vi "PH_Timing.Update GUI.vi"(0 "i ref in":refnum<vi>, 5 "error in (no error)":errorcluster) -> (14 "i ref out":refnum<vi>, 19 "error out":errorcluster)   [LabVIEW 2014, in "PH_Timing.lvlib"]
doc: "By this VI several the blinking of several GUI elements is set which is depending on some information."
uses:
  PH_Timing.lvlib
  PH_Common/PH_Common.lvlib
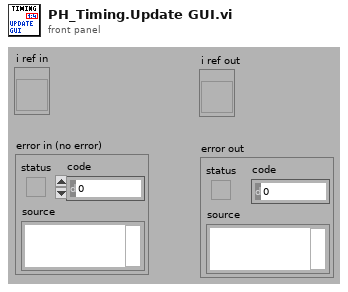
[diagram p1: front panel]
types:
  T1 = typedef "PH_Timing.lvlib/PH_Timing.i attribute.ctl" = cluster{"Sequencer":cluster{"linked?":bool, "Proc State":string, "Ref State":refnum<vi>}, "Gate Generator":cluster{"GD":cluster{"Device Status":T2, "linked?":bool}, "Settings":T3, "GUI Ref":refnum<vi>}, "Interlock Bypass":cluster{"Instancename":string, "Switch linked?":bool, "Device Status":T2, "Ref Status":refnum<vi>}, "Roughtuner":cluster{"Settings":T4, "GUI Ref":refnum<vi>, "GD":cluster{"Device Status":T2, "linked?":bool}}, "0,5Hz Gater":cluster{"Settings":T5, "GUI Ref":refnum<vi>, "GD":cluster{"Device Status":T2, "linked?":bool}}, "Slow Trigger":cluster{"Settings":T6, "GUI Ref":refnum<vi>, "Service ID Delay":i32, "Service ID Ext Trig":i32, "Wanted Settings":T6}, "Timing Mode":cluster{"Mode":T7, "GUI Ref":refnum<vi>, "Service ID T2":i32, "Service ID Mode":i32, "Wanted Mode":T7}, "ns Generator":cluster{"Settings":T8, "ns Generator Settings":refnum<vi>, "GD":cluster{"Device Status":T2, "linked?":bool}}, "Phase FEs":cluster{"Settings":T11, "GUI Ref":refnum<vi>, "Service ID Phase":i32, "Wanted Settings":T11}, "GD GUI Refs":refnum<vi>[], "Heads":T12[], "GUI Ref Delete":refnum<vi>}
  T2 = typedef "PH_StatusHandler.lvlib/PH_StatusHandler.Status.ctl" = i16
  T3 = typedef "PH_Timing.lvlib/PH_Timing.GateGen.ctl" = cluster{"Instance":string, "Channel Gate":i32, "Channel T2":i32, "Width Gate":dbl, "Width T2":dbl, "Delay Gate":dbl, "Delay T2":dbl, "Gate activ":bool, "T2 activ":bool, "System Mode":enum16{"Normal", "Single", "Burst", "Duty Cycle"}}
  T4 = typedef "PH_Timing.lvlib/PH_Timing.Roughtuner.ctl" = cluster{"Instance":string, "Phase PHELIX / UNILAC":cluster{"Channel":u16, "relative to":u16, "Delay [ms]":dbl}, "Pulse Length":cluster{"Channel":u16, "relative to":u16, "Delay [ms]":dbl}, "Trigger":cluster{"externally?":bool, "Rate [Hz]":dbl}}
  T5 = typedef "PH_Timing.lvlib/PH_Timing.0.5HzGater.ctl" = cluster{"Instance":string, "Channel ns FE Delay":i32, "Channel 0.5Hz":i32, "Width ns FE Delay":dbl, "Width 0.5Hz":dbl, "Delay ns FE Delay":dbl, "Delay 0.5Hz":dbl, "ns FE Delay active":bool, "0.5Hz activ":bool, "ns FE Delay inverted":bool, "0.5Hz inverted":bool}
  T6 = typedef "PH_Timing.lvlib/PH_Timing.Slow Trigger Settings.ctl" = cluster{"Delay":dbl, "externally triggered?":bool}
  T7 = typedef "PH_Timing.lvlib/PH_Timing.Timing Mode.ctl" = cluster{"T2":i16, "Modeselector":enum32{"10 Hz", "0.5 Hz", "Shot"}}
  T8 = typedef "PH_Timing.lvlib/PH_Timing.ns Generator.ctl" = cluster{"Instance":string, "Phase fs / ns FE":cluster{"Channel":T9, "Settings":T10}}
  T9 = typedef "Stanford Research DG645 - Driver.lvlib/Channel.ctl" = i32
  T10 = typedef "PH_SRDG645.lvlib/PH_SRDG645.Channel Settings.ctl" = cluster{"Delay [s]":dbl, "relative to":i32}
  T11 = typedef "PH_Timing.lvlib/PH_Timing.Phase FEs.ctl" = cluster{"Phase":dbl}
  T12 = typedef "PH_Timing.lvlib/PH_Timing.PU Data.ctl" = cluster{"linked?":bool, "Data":T13, "GD":cluster{"Device Status":T2, "linked?":bool}, "GUI Ref":refnum<vi>, "PU":T14}
  T13 = typedef "PH_Timing.lvlib/PH_Timing.PU Info.ctl" = cluster{"Act CH?":bool, "GD":string, "CH":i32, "Delay":dbl, "active":bool, "in Use?":bool}
  T14 = typedef "PH_PP_Common.lvlib/PH_PP_Common.PUs.ctl" = enum16{"no Info", "PA-19mm-1", "PA-19mm-2", "PA-45mm-PILC", "PA-45mm-MAIN", "MA-PU-1", "MA-PU-2", "MA-PU-3", "MA-PU-4", "MA-PU-5", "MA-PU-6", "MA-FR", "MA-PILC", "PA-45mm-DP"}
  T15 = cluster{"GD":cluster{"Device Status":T2, "linked?":bool}, "Settings":T3, "GUI Ref":refnum<vi>}
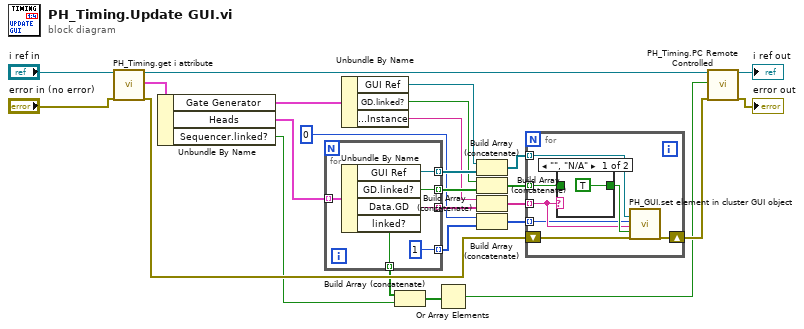
[diagram p0: block diagram]
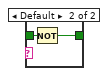
[diagram p2: hidden frame]
diagram:
  n1 = call "PH_Timing.get i attribute.vi"("i ref in"="i ref in", "error in (no error)"="error in (no error)") -> ("i ref out"=w7:refnum<vi>, "i attribute"=w26:T1, "error out"=w10:errorcluster)  [unwired: 15 in]
  n2 = Unbundle By Name(w26) -> ("Gate Generator"=w14:T15, "Heads"=w1:T12[], "Sequencer.linked?"=w4:bool)
  n3 = for {
    tunnel: w1 -> [w32] mode=indexing
    tunnel: [w31] -> w23 mode=indexing
    tunnel: [w30] -> w22 mode=indexing
    tunnel: [w29] -> w21 mode=indexing
    tunnel: [1 ("Cluster index")] -> w20 mode=indexing
    tunnel: [w27] -> w5 mode=indexing
    n4 = Unbundle By Name(w32) -> ("GUI Ref"=w31:refnum<vi>, "GD.linked?"=w30:bool, "Data.GD"=w29:string, "linked?"=w27:bool)
  }
  n5 = Unbundle By Name(w14) -> ("GUI Ref"=w11:refnum<vi>, "GD.linked?"=w12:bool, "Settings.Instance"=w13:string)
  n6 = Build Array (concatenate)(w5, w4) -> (w3:bool[])
  n7 = Or Array Elements(Boolean array=w3) -> (logical OR=w2:bool)
  n8 = Build Array (concatenate)(w11, w23) -> (w19:refnum<vi>[])
  n9 = Build Array (concatenate)(w12, w22) -> (w18:bool[])
  n10 = Build Array (concatenate)(w13, w21) -> (w17:string[])
  n11 = Build Array (concatenate)(0 ("Cluster index"), w20) -> (w16:i32[])
  n12 = for {
    shift-right: [w37] -> w9
    shift-left: w10 -> [w38]
    tunnel: w19 -> [w36] mode=indexing
    tunnel: w18 -> [w35] mode=indexing
    tunnel: w17 -> [w34] mode=indexing
    tunnel: w16 -> [w33] mode=indexing
    n13 = case shown="\"\", \"N/A\"" w34 {
      tunnel: [TRUE ("linked?") w42] -> w39
      tunnel: w35 -> [_ w41]
      frame "", "N/A" {
      }
      frame Default {
        n14 = Not(x=w41) -> (.not. x?=w42:bool)
      }
    }
    n15 = call "PH_GUI.set element in cluster GUI object.vi"("Cluster Ref"=w36, "Cluster index"=w33, "Value"=w34, "Blinking? (false)"=w39, "error in (no error)"=w38) -> ("error out"=w37:errorcluster)  [unwired: 14 in]
  }
  n16 = call "PH_Timing.PC Remote Controlled.vi"("i ref in"=w7, "Remote Controlled?"=w2, "error in (no error)"=w9) -> ("i ref out"=→"i ref out":refnum<vi>, "error out"=→"error out":errorcluster)  [unwired: 15 in]
